vi "binning for loasis TDMS plotter.vi"(8 "y2 col name":string="Bin #", 9 "y1 col name":string="Bin #", 10 "x col name":string="Bin #", 11 "device data Spreadsheet format":string[][](array[string])=[["GOG shot #", "GOG gain", "GOG exposure", "Shot #", "Bin #"], ["1", "0.100000", "0.050000", "1", "1"], ["2", "0.100000", "0.050000", "2", "1"], ["3", "0.100000", "0.050000", "3", "1"], ["4", "0.100000", "0.050000", "4", "1"], ["5", "0.100000", "0.050000", "5", "1"], ["6", "0.130000", "0.050000", "6", "2"], ["7", "0.130000", "0.050000", "7", "2"], ["8", "0.130000", "0.050000", "8", "2"], ["9", "0.130000", "0.050000", "9", "2"], ["10", "0.130000", "0.050000", "10", "2"], ["11", "0.160000", "0.050000", "11", "3"], ["12", "0.160000", "0.050000", "12", "3"], ["13", "0.160000", "0.050000", "13", "3"], ["14", "0.160000", "0.050000", "14", "3"], ["15", "0.160000", "0.050000", "15", "3"], ["16", "0.190000", "0.050000", "16", "4"], ["17", "0.190000", "0.050000", "17", "4"], ["18", "0.190000", "0.050000", "18", "4"], ["19", "0.190000", "0.050000", "19", "4"], ["20", "0.190000", "0.050000", "20", "4"]]) -> (3 "xy graph bin":cluster{dbl[], dbl[]}[](graph)=[{[5.5, 15.5, 25.5, 35.5, 45.5, 55.5, 0.0], [0.1, 0.1, 0.15, 0.15, 0.2, 0.2, 0.0]}, {[5.5, 5.5, nan, 15.5, 15.5, nan, 25.5, 25.5, nan, 35.5, 35.5, nan, 45.5, 45.5, nan, 55.5, 55.5, nan, 0.0, 0.0, nan], [0.1, 0.1, nan, 0.1, 0.1, nan, 0.15, 0.15, nan, 0.15, 0.15, nan, 0.2, 0.2, nan, 0.2, 0.2, nan, 0.0, 0.0, nan]}, {[5.5, 15.5, 25.5, 35.5, 45.5, 55.5, 0.0], [5.5, 15.5, 25.5, 35.5, 45.5, 55.5, 0.0]}, {[5.5, 5.5, nan, 15.5, 15.5, nan, 25.5, 25.5, nan, 35.5, 35.5, nan, 45.5, 45.5, nan, 55.5, 55.5, nan, 0.0, 0.0, nan], [3.0, 8.0, nan, 13.0, 18.0, nan, 23.0, 28.0, nan, 33.0, 38.0, nan, 43.0, 48.0, nan, 53.0, 58.0, nan, 0.0, 0.0, nan]}])   [LabVIEW 2013]
panel:
  out "Means":dbl[](array[numeric])
  out "Col titles":string[](array[string])
  out "bin values":string[](array[string])
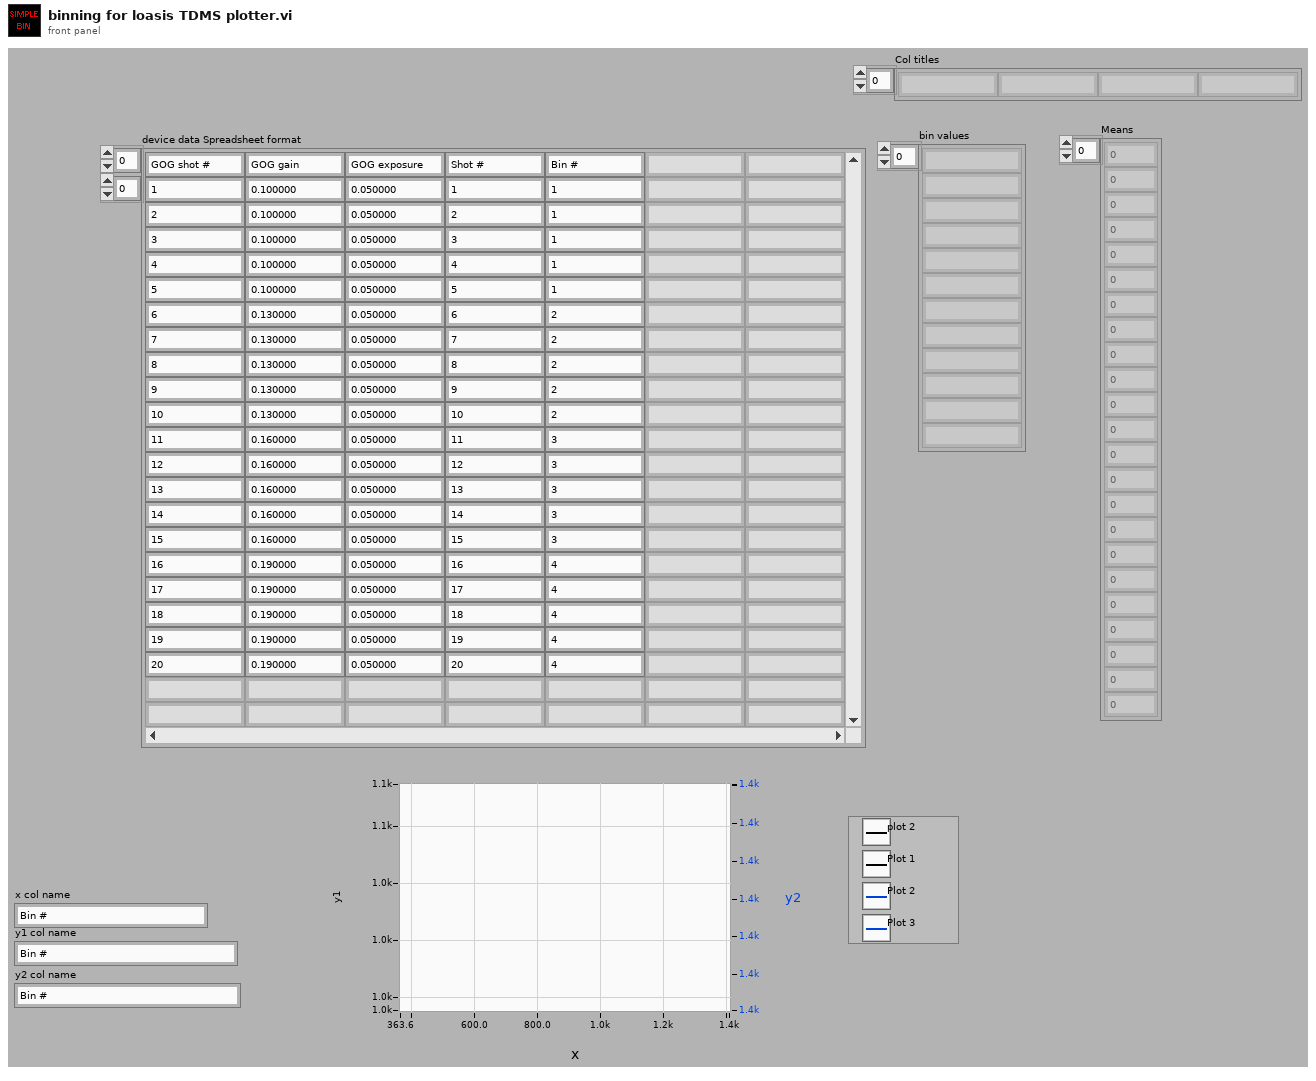
[diagram p1: front panel]
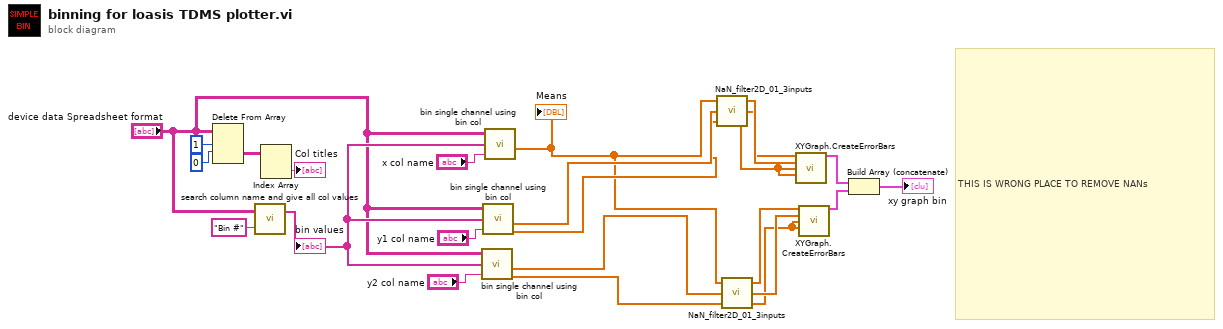
[diagram p0: block diagram]
diagram:
  # "THIS IS WRONG PLACE TO REMOVE NANs"
  n1 = Delete From Array(array="device data Spreadsheet format", length=1, index (row)=0) -> (deleted portion=w21:string[][])  [unwired: 1 in, 1 out]
  n2 = call "search column name and give all col values.vi"("column name to get"="Bin #", "input 2d array"="device data Spreadsheet format") -> ("column values"=w14:string[])  [unwired: 1 out]
  "bin values" <- w14
  n3 = Index Array(array=w21) -> (element=→"Col titles":string[])  [unwired: 2 in]
  n4 = call "bin single channel using bin col.vi"("device data Spreadsheet format"="device data Spreadsheet format", "bin values"=w14, "col name"="y2 col name") -> ("Means"=w4:dbl[], "Sds"=w2:dbl[])  [unwired: 2 out]
  n5 = call "bin single channel using bin col.vi"("device data Spreadsheet format"="device data Spreadsheet format", "bin values"=w14, "col name"="y1 col name") -> ("Means"=w11:dbl[], "Sds"=w10:dbl[])  [unwired: 2 out]
  n6 = call "bin single channel using bin col.vi"("device data Spreadsheet format"="device data Spreadsheet format", "bin values"=w14, "col name"="x col name") -> ("Means"=w6:dbl[])  [unwired: 3 out]
  "Means" <- w6
  n7 = call "NaN_filter2D_01_3inputs.vi"("Error in"=w10, "Yin"=w11, "Xin"=w6) -> ("error out"=w7:dbl[], "Xout"=w8:dbl[], "Yout"=w9:dbl[])
  n8 = call "NaN_filter2D_01_3inputs.vi"("Error in"=w2, "Yin"=w4, "Xin"=w6) -> ("error out"=w1:dbl[], "Xout"=w3:dbl[], "Yout"=w5:dbl[])
  n9 = call "XYGraph.CreateErrorBars.vi"("X"=w8, "Y"=w9, "error low"=w7, "error high"=w7) -> ("xy graph bin 2"=w18:cluster{"X":dbl[], "Y":dbl[]}[])  [unwired: 11 out]
  n10 = call "XYGraph.CreateErrorBars.vi"("X"=w5, "Y"=w3, "error low"=w1, "error high"=w1) -> ("xy graph bin 2"=w20:cluster{"X":dbl[], "Y":dbl[]}[])  [unwired: 11 out]
  n11 = Build Array (concatenate)(w18, w20) -> (→"xy graph bin":cluster{"X":dbl[], "Y":dbl[]}[])
